vi "Create Instance Impl.vi"(8 "error in (no error)":errorcluster, 10 "Stage Configuration":T1={"Serial Port"="COM4", "Forward Step (mm)"=0.4, "Lane Length (mm)"=6.0, "Lane Separation (mm)"=0.8, "Stage Type"=enum."Ti2", "Autofocus Z Planes"=9, "Autofocus Range (um)"=30.0, "Stage Limits"={"Y Min"=-4.5, "Y Max"=3.0, "X Min"=-19.0, "X Max"=33.5}, "Slide (mm)"={"top"=-13.0, "right"=-22.3, "width"=60.0, "height"=25.4}}, 11 "Stage Controller in":refnum<class "Stage Controller.lvclass">) -> (0 "error out":errorcluster, 3 "Stage Controller out":refnum<class "Stage Controller.lvclass">)   [LabVIEW 2023, in "Stage Controller.lvlib" / "Stage Controller.lvclass"]
uses:
  Stage Controller.lvclass
  Stage Controller.lvclass/Stage Controller.ctl
  Resources/Type Defs/Stage Configuration.ctl
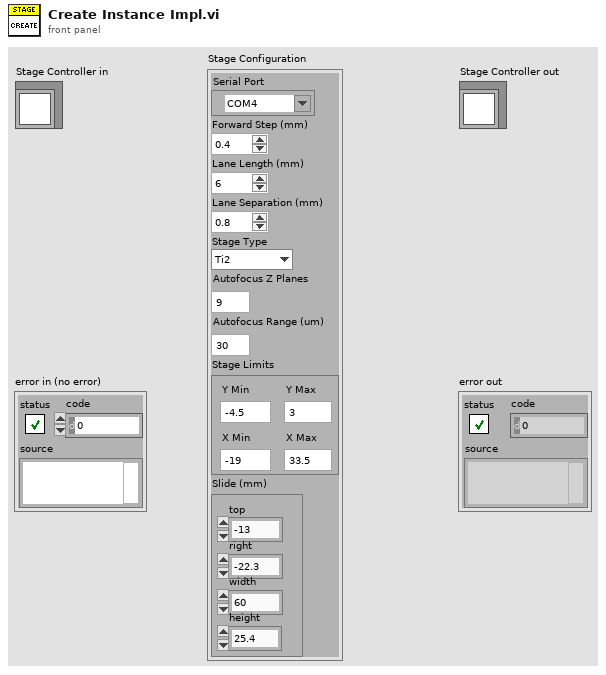
[diagram p1: front panel]
types:
  T1 = typedef "Stage Configuration.ctl" = cluster{"Serial Port":refnum<visa-resource-name>, "Forward Step (mm)":dbl, "Lane Length (mm)":dbl, "Lane Separation (mm)":dbl, "Stage Type":enum16{"Disabled", "ESP301", "Ti2", "Ludl", "ASI"}, "Autofocus Z Planes":i32, "Autofocus Range (um)":dbl, "Stage Limits":cluster{"Y Min":dbl, "Y Max":dbl, "X Min":dbl, "X Max":dbl}, "Slide (mm)":cluster{"top":dbl, "right":dbl, "width":dbl, "height":dbl}}
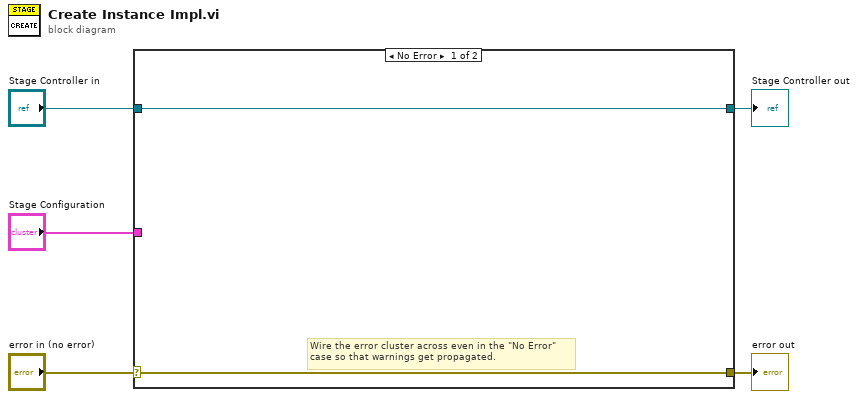
[diagram p0: block diagram]
diagram:
  n1 = case shown="No Error" "error in (no error)" {
    selector: "error in (no error)" -> [w6 w9]
    tunnel: [w6 w9] -> w4
    tunnel: [w7 w8] -> w2
    tunnel: "Stage Controller in" -> [w7 w8]
    tunnel: "Stage Configuration" -> [_ _]
    frame No Error {
      # "Wire the error cluster across even in the \"No Error\"\ncase so that warnings get propagated."
    }
    frame Error {
    }
  }
  "error out" <- w4
  "Stage Controller out" <- w2
